vi "collectCI_tt.vi"() -> (1 "size(s)":i32)   [LabVIEW 2015]
uses:
  <vilib>/DAQmx/read.llb/DAQmx Read (Counter 1D U32 1Chan NSamp).vi
  <vilib>/DAQmx/miscellaneous.llb/DAQmx Fill In Error Info.vi
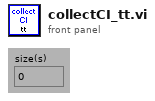
[diagram p1: front panel]
types:
  T1 = typedef "LVRectTypeDef.ctl" = cluster{"Left":i16, "Top":i16, "Right":i16, "Bottom":i16}
  T2 = cluster{"Xpixels":i32, "Vxminref":dbl, "Vxmaxref":dbl, "P":dbl, "Ypixels":i32, "Vyminref":dbl, "Vymaxref":dbl, "srate":sgl, "sAOxy":i32, "timeout":dbl, "type":string, "date":string, "time":string, "Colormap":u16, "Drawing Mode":u16, "Scanning Mode":u16, "square pixels":bool, "square matrix":bool, "Xpixels Img":i32, "Vx-min Img":dbl, "VX-max Img":dbl, "Ypixels Img":i32, "Vy-min Img":dbl, "Vy-max Img ":dbl, "Angle Img":dbl, "autoshutter":bool, "finite":bool, "cont":bool, "wavdet":bool, "measpoints":i32, "avpp":i32, "bufferAO":i32, "bufferAI":i32, "starttick":u32, "waveform":path, "Vx-ref":dbl, "Vy-ref":dbl, "refreshrate":dbl, "refreshbuffer":i32, "tt_cycles":i32, "motorref":refnum<k7>, "mirrorswitch":refnum<k7>, "sample mode":i32, "maxbufferAI":i32, "srateAODO":sgl, "bin":sgl, "Pel":sgl, "Angle draw":dbl, "srate Img":sgl, "ROIimg_plotbounds":T1, "auto OD":bool, "ODfilt":u16, "aAI":i32[], "aCI":i32[], "aAO":u32[], "aDO":u32[], "refwfsize":dbl, "Lifetime":bool, "Vz-Img":dbl, "Vz-ref":dbl, "Vz-reset":dbl, "AIoverride":bool, "aAS":u32[], "XYZstart":dbl[]}
  T3 = cluster{"CI":refnum<k21>[], "E_CI":errorcluster[]}
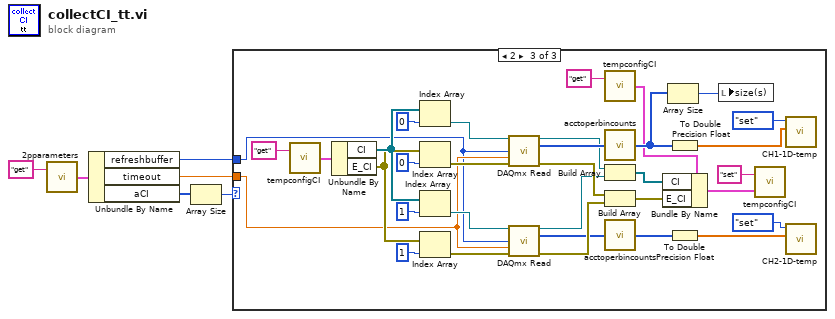
[diagram p0: block diagram]
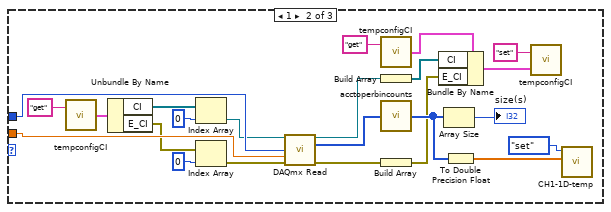
[diagram p3: hidden frame]
diagram:
  n1 = call "2pparameters.vi"("command"="get") -> ("params out"=w6:T2)  [unwired: 1 in]
  n2 = Unbundle By Name(w6) -> ("refreshbuffer"=w1:i32, "timeout"=w2:dbl, "aCI"=w3:i32[])
  n3 = Array Size(array=w3) -> (size(s)=w4:i32)
  n4 = case shown="2" w4 {
    tunnel: w2 -> [_ w21 w37]
    tunnel: w1 -> [_ w20 w36]
    frame 0, Default {
    }
    frame 1 {
      n5 = call "tempconfigCI.vi"("command"="get") -> ("Temp Config out"=w18:T3)  [unwired: 1 in]
      n6 = Unbundle By Name(w18) -> ("CI"=w16:refnum<k21>[], "E_CI"=w15:errorcluster[])
      n7 = Index Array(array=w16, index=0) -> (element=w13:refnum<k21>)
      n8 = Index Array(array=w15, index=0) -> (element=w12:errorcluster)
      n9 = call-poly <vilib>:"DAQmx Read.vi"("task/channels in"=w13, "number of samples per channel"=w20, "timeout"=w21, "error in"=w12) -> ("task out"=w11:refnum<k21>, "data"=w27:u32[], "error out"=w9:errorcluster)  [unwired: 9 in]
      n10 = call "tempconfigCI.vi"("command"="get") -> ("Temp Config out"=w22:T3)  [unwired: 1 in]
      n11 = Build Array(w11) -> (w10:refnum<k21>[])
      n12 = call "acctoperbincounts.vi"("accumulative counts"=w27) -> ("counts per bin"=w26:u32[])
      n13 = Build Array(w9) -> (w8:errorcluster[])
      n14 = Bundle By Name(cluster=w22, "CI"=w10, "E_CI"=w8) -> (w25:T3)
      n15 = Array Size(array=w26) -> (size(s)=→"size(s)":i32)
      n16 = To Double Precision Float(number=w26) -> (double precision float=w28:dbl[])
      n17 = call "tempconfigCI.vi"("Temp Config in"=w25, "command"="set") -> ()  [unwired: 1 out]
      n18 = call "CH1-1D-temp.vi"("array in"=w28, "command"=enum16{"get", "set", "clear", "append"}."set") -> ()  [unwired: 2 in, 2 out]
    }
    frame 2 {
      n19 = call "tempconfigCI.vi"("command"="get") -> ("Temp Config out"=w53:T3)  [unwired: 1 in]
      n20 = Unbundle By Name(w53) -> ("CI"=w41:refnum<k21>[], "E_CI"=w40:errorcluster[])
      n21 = Index Array(array=w41, index=0) -> (element=w50:refnum<k21>)
      n22 = Index Array(array=w40, index=0) -> (element=w49:errorcluster)
      n23 = Index Array(array=w41, index=1) -> (element=w39:refnum<k21>)
      n24 = Index Array(array=w40, index=1) -> (element=w38:errorcluster)
      n25 = call-poly <vilib>:"DAQmx Read.vi"("task/channels in"=w50, "number of samples per channel"=w36, "timeout"=w37, "error in"=w49) -> ("task out"=w48:refnum<k21>, "data"=w60:u32[], "error out"=w46:errorcluster)  [unwired: 9 in]
      n26 = call-poly <vilib>:"DAQmx Read.vi"("task/channels in"=w39, "number of samples per channel"=w36, "timeout"=w37, "error in"=w38) -> ("task out"=w34:refnum<k21>, "data"=w30:u32[], "error out"=w35:errorcluster)  [unwired: 9 in]
      n27 = call "tempconfigCI.vi"("command"="get") -> ("Temp Config out"=w55:T3)  [unwired: 1 in]
      n28 = call "acctoperbincounts.vi"("accumulative counts"=w60) -> ("counts per bin"=w59:u32[])
      n29 = Build Array(w48, w34) -> (w47:refnum<k21>[])
      n30 = Build Array(w46, w35) -> (w45:errorcluster[])
      n31 = call "acctoperbincounts.vi"("accumulative counts"=w30) -> ("counts per bin"=w33:u32[])
      n32 = Bundle By Name(cluster=w55, "CI"=w47, "E_CI"=w45) -> (w58:T3)
      n33 = Array Size(array=w59) -> (size(s)=w44:i32)
      n34 = To Double Precision Float(number=w59) -> (double precision float=w61:dbl[])
      n35 = To Double Precision Float(number=w33) -> (double precision float=w32:dbl[])
      n36 = local write "size(s)"(w44) -> ()
      n37 = call "tempconfigCI.vi"("Temp Config in"=w58, "command"="set") -> ()  [unwired: 1 out]
      n38 = call "CH1-1D-temp.vi"("array in"=w61, "command"=enum16{"get", "set", "clear", "append"}."set") -> ()  [unwired: 2 in, 2 out]
      n39 = call "CH2-1D-temp.vi"("array in"=w32, "command"=enum16{"get", "set", "clear", "append"}."set") -> ()  [unwired: 2 in, 2 out]
    }
  }
